vi "Test_BME280.vi"() -> ()   [LabVIEW 2014]
uses:
  BME280_class/TrimmingParameters.ctl
  <vilib>/MakerHub/LINX/Public/Utilities/Open Local.vi
  BME280_class/BME280.lvclass
  <vilib>/MakerHub/LINX/LMH-LINX.lvlib
panel:
  out "Boolean":bool
  in  "stop 2":bool
  out "TrimmingParameters":T1
  out "Pressure":dbl
  out "Data 2":u8[](array[numeric])
  out "RH":dbl
  out "Lynx Setup error":errorcluster
  out "Data":u8[](array[numeric])
  in  "stop":bool
  out "Temperature":dbl
  out "Error Out":errorcluster
  out "Device Name":string
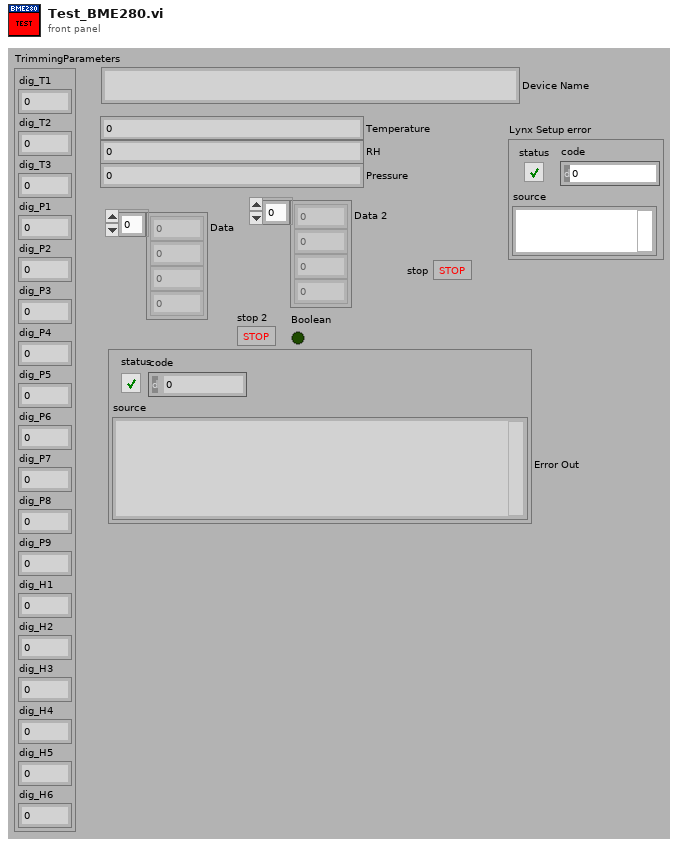
[diagram p1: front panel]
types:
  T1 = typedef "BME280.lvclass/TrimmingParameters.ctl" = cluster{"dig_T1":u16, "dig_T2":i16, "dig_T3":i16, "dig_P1":u16, "dig_P2":i16, "dig_P3":i16, "dig_P4":i16, "dig_P5":i16, "dig_P6":i16, "dig_P7":i16, "dig_P8":i16, "dig_P9":i16, "dig_H1":u8, "dig_H2":i16, "dig_H3":u8, "dig_H4":i16, "dig_H5":i16, "dig_H6":i8}
  T2 = typedef "LMH-LINX.lvlib/LINX Ref.ctl" = cluster{"IO":T3, "Interface":T4, "LINX Device Config":T5}
  T3 = typedef "LMH-LINX.lvlib/Platform.ctl" = enum16{"Remote", "Local"}
  T4 = typedef "LMH-LINX.lvlib/Interface.ctl" = enum16{"Serial", "TCP"}
  T5 = typedef "LMH-LINX.lvlib/Device.lvlib/LINX Device Config.ctl" = cluster{"Interface":T4, "COM Port":refnum<visa-resource-name>, "TCP Configuration":T6, "Device Family":u8, "Device ID":u8, "Device Name":string, "TCP Ref":refnum<k5>, "Channels":T7}
  T6 = typedef "LMH-LINX.lvlib/Device.lvlib/TCP Config.ctl" = cluster{"IP Address":string, "Port":u16}
  T7 = typedef "LMH-LINX.lvlib/Channels.ctl" = cluster{"DI":u8[], "DO":u8[], "AI":u8[], "AO":u8[], "PWM":u8[], "QE":u8[], "UART":u8[], "I2C 2":u8[], "SPI":u8[], "CAN":u8[], "Servo":u8[], "AI Ref (V)":dbl, "AI Resolution (Bits)":u8, "AO Ref (V)":dbl, "AO Resolution (Bits)":u8}
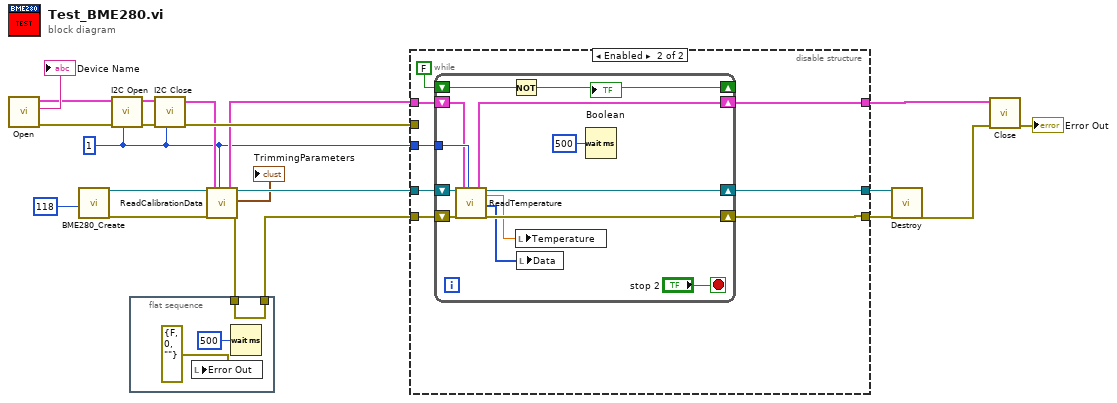
[diagram p0: block diagram]
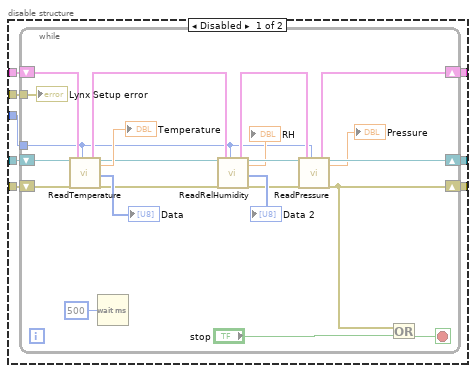
[diagram p2: hidden frame]
diagram:
  w1 = u8 1 ("I2C Channel (0)")
  n1 = call-poly <vilib>:"Open.vi"() -> ("Error Out"=w9:errorcluster, "Device Name"=→"Device Name":string, "LINX Resource"=w12:T2)  [unwired: 9 in]
  n2 = call "BME280_Create.vi"("I2C Slave Address (0)"=u8 118) -> ("reference out"=w13:refnum<class "BME280.lvclass">, "error out"=w6:errorcluster)  [unwired: 17 in]
  n3 = call <vilib>:"I2C Open.vi"("I2C Channel (0)"=w1, "Error In"=w9, "LINX Resource"=w12) -> ("Error Out"=w10:errorcluster, "LINX Resource"=w11:T2)  [unwired: 7 in]
  n4 = flat-sequence {
    tunnel: [w23] -> w15
    tunnel: w5 -> [w23]
    frame #0 {
      n5 = local write "Error Out"(errorcluster {"status"=FALSE, "code"=0, "source"=""} ("Error Out")) -> ()
      n6 = Wait (ms)(milliseconds to wait=u32 500) -> ()  [unwired: 1 out]
    }
  }
  n7 = call <vilib>:"I2C Close.vi"("I2C Channel (0)"=w1, "Error In"=w10, "LINX Resource"=w11) -> ("Error Out"=w8:errorcluster, "LINX Resource"=w4:T2)  [unwired: 7 in]
  n8 = call-dynamic "ReadCalibrationData.vi"("reference in"=w13, "error in (no error)"=w6, "LINX Resource"=w4, "I2C Channel (0)"=w1) -> ("LINX Resource"=w3:T2, "reference out"=w7:refnum<class "BME280.lvclass">, "TrimmingParameters"=→"TrimmingParameters":T1, "error out"=w5:errorcluster)  [unwired: 12 in]
  n9 = disable-structure shown="Enabled" {
    disable-tunnel: [w32 w59] -> w21
    disable-tunnel: [w31 w60] -> w20
    disable-tunnel: w15 -> [w30 w62]
    disable-tunnel: [w29 w56] -> w14
    disable-tunnel: w8 -> [w28 _]
    disable-tunnel: w7 -> [w27 w61]
    disable-tunnel: w3 -> [w26 w57]
    disable-tunnel: w1 -> [w25 w58]
    frame Disabled {
      n10 = while {
        shift-right: [w39] -> w32
        shift-left: w27 -> [w51]
        shift-right: [w37] -> w31
        shift-left: w30 -> [w50]
        shift-right: [w34] -> w29
        shift-left: w26 -> [w49]
        tunnel: w28 -> [w52]
        tunnel: w25 -> [w33]
        stop <- w53 stop-if-true
        n11 = call-dynamic "ReadTemperature.vi"("reference in"=w51, "error in (no error)"=w50, "LINX Resource"=w49, "I2C Channel (0)"=w33) -> ("LINX Resource"=w42:T2, "reference out"=w45:refnum<class "BME280.lvclass">, "Temperature"=→"Temperature":dbl, "Data Temp"=→"Data":u8[], "error out"=w44:errorcluster)  [unwired: 11 in]
        n12 = Wait (ms)(milliseconds to wait=u32 500) -> ()  [unwired: 1 out]
        n13 = call-dynamic "ReadRelHumidity.vi"("reference in"=w45, "error in (no error)"=w44, "LINX Resource"=w42, "I2C Channel (0)"=w33) -> ("LINX Resource"=w35:T2, "reference out"=w43:refnum<class "BME280.lvclass">, "RH"=→"RH":dbl, "Data RH"=→"Data 2":u8[], "error out"=w38:errorcluster)  [unwired: 11 in]
        n14 = call-dynamic "ReadPressure.vi"("reference in"=w43, "error in (no error)"=w38, "LINX Resource"=w35, "I2C Channel (0)"=w33) -> ("LINX Resource"=w34:T2, "reference out"=w39:refnum<class "BME280.lvclass">, "Pressure"=→"Pressure":dbl, "error out"=w37:errorcluster)  [unwired: 11 in, 1 out]
        n15 = Or(x=w37, y="stop") -> (x .or. y?=w53:bool)
        "Lynx Setup error" <- w52
      }
    }
    frame Enabled {
      n16 = while {
        tunnel: w58 -> [w71]
        shift-right: [w73] -> w60
        shift-left: w62 -> [w75]
        shift-right: [w72] -> w59
        shift-left: w61 -> [w74]
        shift-right: [w69] -> w56
        shift-left: w57 -> [w70]
        shift-right: [w63] -> _
        shift-left: FALSE ("Boolean") -> [w64]
        stop <- "stop 2" stop-if-true
        n17 = call-dynamic "ReadTemperature.vi"("reference in"=w74, "error in (no error)"=w75, "LINX Resource"=w70, "I2C Channel (0)"=w71) -> ("LINX Resource"=w69:T2, "reference out"=w72:refnum<class "BME280.lvclass">, "Temperature"=w68:dbl, "Data Temp"=w67:u8[], "error out"=w73:errorcluster)  [unwired: 11 in]
        n18 = Not(x=w64) -> (.not. x?=w63:bool)
        "Boolean" <- w63
        n19 = local write "Temperature"(w68) -> ()
        n20 = local write "Data"(w67) -> ()
        n21 = Wait (ms)(milliseconds to wait=u32 500) -> ()  [unwired: 1 out]
      }
    }
  }
  n22 = call-dynamic "Destroy.vi"("reference in"=w21, "error in (no error)"=w20) -> ("error out"=w18:errorcluster)  [unwired: 16 in, 1 out]
  n23 = call <vilib>:"Close.vi"("Error In"=w18, "LINX Resource"=w14) -> ("Error Out"=→"Error Out":errorcluster)  [unwired: 9 in]
